vi "Visualise FFT.vi"(6 "Frequency Metedata":T2, 8 "error in (no error)":errorcluster, 9 "Signal Density Plot":T3, 10 "FFT Data":T1, 11 "UI Root in":refnum<class "UI Root.lvclass">) -> (0 "error out":errorcluster, 3 "UI Root out":refnum<class "UI Root.lvclass">)   [LabVIEW 2020, in "UI Root.lvlib" / "UI Root.lvclass"]
uses:
  UI Root.lvclass
  Signal Density Plot Data.ctl
  <vilib>/Utility/miscctls.llb/LVOffsetAndMultiplierTypeDef.ctl
  Frequency Metadata.ctl
  FFT Plot Data.ctl
  UI Root.lvclass/UI Root.ctl
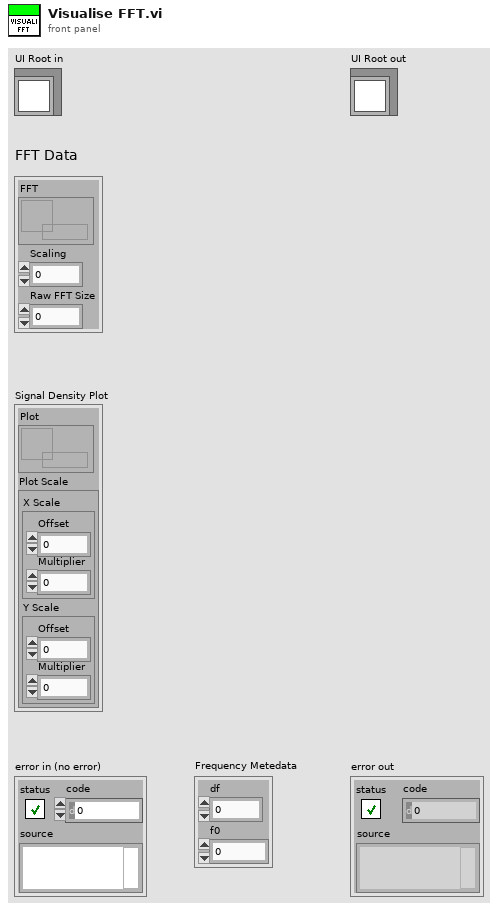
[diagram p1: front panel]
types:
  T1 = typedef "UI Root.lvlib/UI Root.lvclass/FFT Plot Data.ctl" = cluster{"FFT":refnum<data-value>, "Scaling":dbl, "Raw FFT Size":i32}
  T2 = typedef "UI Root.lvlib/UI Root.lvclass/Frequency Metadata.ctl" = cluster{"df":dbl, "f0":dbl}
  T3 = typedef "UI Root.lvlib/UI Root.lvclass/Signal Density Plot Data.ctl" = cluster{"Plot":refnum<data-value>, "Plot Scale":cluster{"X Scale":T4, "Y Scale":T4}}
  T4 = typedef "LVOffsetAndMultiplierTypeDef.ctl" = cluster{"Offset":dbl, "Multiplier":dbl}
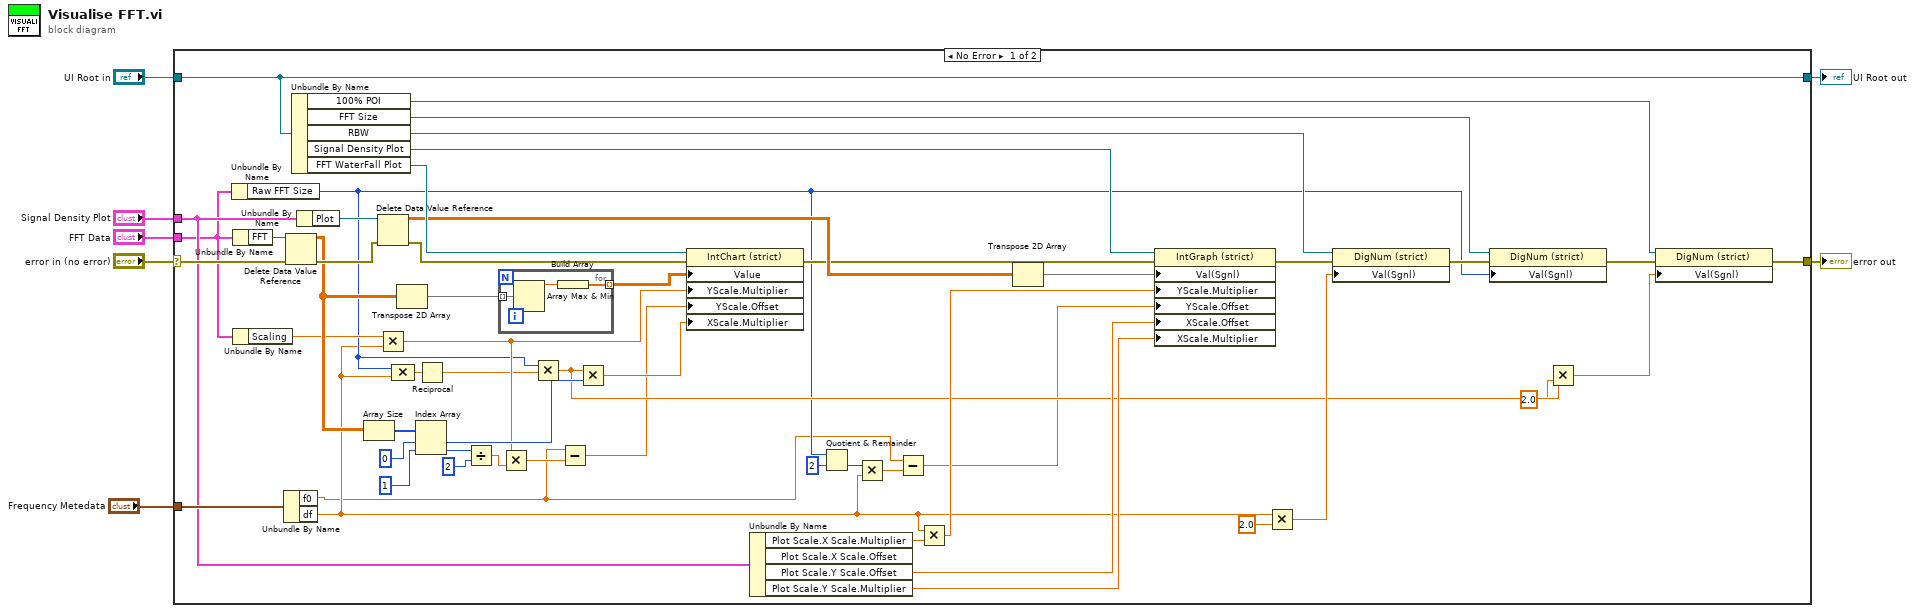
[diagram p0: block diagram]
diagram:
  n1 = case shown="No Error" "error in (no error)" {
    selector: "error in (no error)" -> [w60 w66]
    tunnel: [w22 w66] -> w6
    tunnel: [w61 w65] -> w4
    tunnel: "UI Root in" -> [w61 w65]
    tunnel: "FFT Data" -> [w29 _]
    tunnel: "Signal Density Plot" -> [w53 _]
    tunnel: "Frequency Metedata" -> [w54 _]
    frame No Error {
      n2 = Unbundle By Name(w29) -> ("Raw FFT Size"=w14:i32)
      n3 = Unbundle By Name(w29) -> ("FFT"=w47:refnum<data-value>)
      n4 = Unbundle By Name(w29) -> ("Scaling"=w28:dbl)
      n5 = Unbundle By Name(w54) -> ("f0"=w9:dbl, "df"=w11:dbl)
      n6 = Delete Data Value Reference(data value reference=w47, error in=w60) -> (data value=w33:sgl[][], error out=w58:errorcluster)
      n7 = Unbundle By Name(w61) -> ("100% POI"=w21:refnum<vi>, "FFT Size"=w34:refnum<vi>, "RBW"=w39:refnum<vi>, "Signal Density Plot"=w59:refnum<vi>, "FFT WaterFall Plot"=w57:refnum<vi>)
      n8 = Unbundle By Name(w53) -> ("Plot"=w55:refnum<data-value>)
      n9 = Array Size(array=w33) -> (size(s)=w41:i32[])
      n10 = Delete Data Value Reference(data value reference=w55, error in=w58) -> (data value=w49:sgl[][], error out=w56:errorcluster)
      n11 = Multiply(x=w28, y=w11) -> (x*y=w24:dbl)
      n12 = Compound Arithmetic op=MULTIPLY(w14, w11) -> (w27:dbl)
      n13 = Transpose 2D Array(2D array=w33) -> (transposed array=w32:sgl[][])
      n14 = Index Array(array=w41, index #1=0 ("index"), index #2=1 ("index")) -> (element #1=w25:i32, element #2=w35:i32)
      n15 = Reciprocal(x=w27) -> (1/x=w20:dbl)
      n16 = Divide(x=w35, y=2) -> (x/y=w45:dbl)
      n17 = for {
        tunnel: w32 -> [w64] mode=indexing
        tunnel: [w62] -> w31 mode=indexing
        n18 = Array Max & Min(array=w64) -> (max value=w63:sgl)  [unwired: 3 out]
        n19 = Build Array(w63) -> (w62:sgl[])
      }
      n20 = Multiply(x=w24, y=w45) -> (x*y=w44:dbl)
      n21 = Multiply(x=w14, y=w20) -> (x*y=w18:dbl)
      n22 = Subtract(x=w9, y=w44) -> (x-y=w15:dbl)
      n23 = Multiply(x=w18, y=w25) -> (x*y=w19:dbl)
      n24 = property class="IntChart (strict)"(reference=w57, error in=w56, "Value"=w31, "YScale.Multiplier"=w24, "YScale.Offset"=w15, "XScale.Multiplier"=w19) -> (error out=w42:errorcluster)  [unwired: 1 out]
      n25 = Unbundle By Name(w53) -> ("Plot Scale.X Scale.Multiplier"=w52:dbl, "Plot Scale.Y Scale.Offset"=w50:dbl, "Plot Scale.Y Scale.Multiplier"=w51:dbl)  [unwired: 1 out]
      n26 = Quotient & Remainder(x=w14, y=2) -> (floor(x/y)=w12:i32)  [unwired: 1 out]
      n27 = Multiply(x=w12, y=w11) -> (x*y=w10:dbl)
      n28 = Subtract(x=w9, y=w10) -> (x-y=w8:dbl)
      n29 = Multiply(x=w11, y=w52) -> (x*y=w48:dbl)
      n30 = Transpose 2D Array(2D array=w49) -> (transposed array=w30:sgl[][])
      n31 = property class="IntGraph (strict)"(reference=w59, error in=w42, "Val(Sgnl)"=w30, "YScale.Multiplier"=w48, "YScale.Offset"=w8, "XScale.Offset"=w50, "XScale.Multiplier"=w51) -> (error out=w38:errorcluster)  [unwired: 1 out]
      n32 = Multiply(x=w11, y=2.0) -> (x*y=w37:dbl)
      n33 = property class="DigNum (strict)"(reference=w39, error in=w38, "Val(Sgnl)"=w37) -> (error out=w36:errorcluster)  [unwired: 1 out]
      n34 = property class="DigNum (strict)"(reference=w34, error in=w36, "Val(Sgnl)"=w14) -> (error out=w23:errorcluster)  [unwired: 1 out]
      n35 = Multiply(x=w18, y=2.0) -> (x*y=w16:dbl)
      n36 = property class="DigNum (strict)"(reference=w21, error in=w23, "Val(Sgnl)"=w16) -> (error out=w22:errorcluster)  [unwired: 1 out]
    }
    frame Error {
    }
  }
  "error out" <- w6
  "UI Root out" <- w4
